vi "integral_ctrl_v7.vi"(4 "Lower limit":fxp<+/-,25,4>=-5.0, 5 "Upper limit":fxp<+/-,25,4>=5.0, 7 "Enable?":bool, 10 "Ki*Ts":fxp<+,16,0>, 11 "Input":fxp<+/-,25,4>) -> (3 "Output":fxp<+/-,25,4> format="%.23g")   [LabVIEW 2017, in "FPGA Controllers.lvlib"]
doc: "Integral controller implementation\nImplements: Ki/s in discrete time. (Ki*Ts) z / (z-1)\n\nAnti-windup limits can be specified as needed."
uses:
  FPGA Controllers.lvlib
  <vilib>/rvi/FXPMathLib/FxpMul/XNode/nifxpmath_Multiplier.xnode
  <vilib>/rvi/FXPMathLib/FxpAdd/XNode/nifxpmath_Add.xnode
  <vilib>/Platform/TimedLoop/XDataNode/XDataNode.xnode
  <vilib>/Platform/TimedLoop/XDataNode/nitl_modes.ctl
  <vilib>/Platform/TimedLoop/XDataNode/XDNodeRunTimeDep.lvlib
  <vilib>/Platform/TimedLoop/XDataNode/wakeup.ctl
  <vilib>/Platform/TimedLoop/XDataNode/timing_clust.ctl
  <vilib>/rvi/FXPMathLib/sim/FxpSim.dll
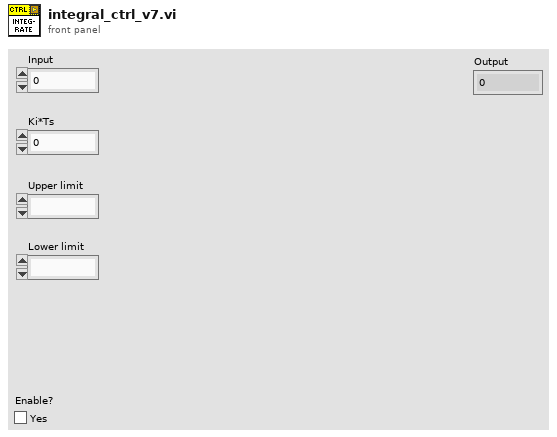
[diagram p1: front panel]
types:
  T1 = typedef "XDNodeRunTimeDep.lvlib/timing_clust.ctl" = cluster{"Expected End [f-1]":u64, "Actual End [f-1]":u64, "Finished Late? [f-1]":bool, "Expected End [i-1]":u64, "Actual End [i-1]":u64, "Finished Late? [i-1]":bool, "Expected Start [i]":u64, "Actual Start [i]":u64, "Expected Start [f]":u64, "Actual Start [f]":u64, "Source Name":string, "Structure Name":string, "Period":i64, "Deadline":i64, "Offset":i64, "Start":i64, "Priority":i32, "Timeout":i32, "Mode":T2, "Wakeup Reason":T3, "Error":errorcluster, "Source Type":string, "Secondary Source Type":string, "Global End Time":u64, "Global Start Time":u64, "Frame Duration":u64, "Iteration Duration":u64, "Assigned CPU":i32, "I/O Scan Engine Mode":u32}
  T2 = typedef "XDNodeRunTimeDep.lvlib/nitl_modes.ctl" = enum32{"No Change", "Process missed periods, maintain original phase", "Discard missed periods, maintain original phase", "Process missed periods, ignore original phase", "Discard missed periods, ignore original phase"}
  T3 = typedef "XDNodeRunTimeDep.lvlib/wakeup.ctl" = enum32{"Normal", "Aborted", "Asynchronous wakeup", "Timing source error", "Timed loop error", "Timeout"}
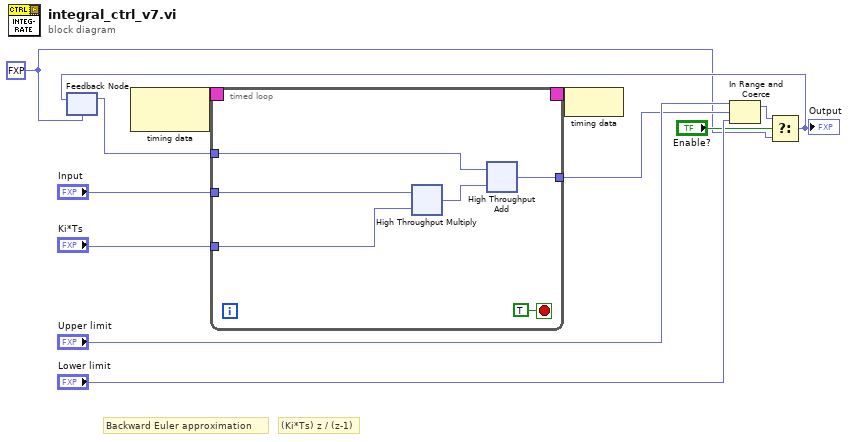
[diagram p0: block diagram]
diagram:
  w2 = fxp<+/-,25,4> 0.0 ("Input")
  # "(Ki*Ts) z / (z-1)"
  # "Backward Euler approximation"
  n1 = feedback #1(w2) -> (w4:fxp<+/-,25,4>)
  n2 = node-c288() -> (w6:T1)  [unwired: 1 in]
  n3 = timed-loop {
    timing: w6 -> [_]
    timing-out: [_] -> w5
    tunnel: "Ki*Ts" -> [w13]
    tunnel: w4 -> [w17]
    tunnel: "Input" -> [w18]
    tunnel: [w16] -> w7
    stop <- TRUE stop-if-true
    n4 = xnode ("High Throughput Multiply")("x"=w18, "y"=w13) -> ("x*y"=w15:fxp<+/-,25,4>)
    n5 = xnode ("High Throughput Add")("x"=w17, "y"=w15) -> ("x+y"=w16:fxp<+/-,25,4>)
  }
  n6 = node-c288(w5) -> ()
  n7 = In Range and Coerce(upper limit="Upper limit", x=w7, lower limit="Lower limit") -> (coerced(x)=w1:fxp<+/-,25,4>)  [unwired: 1 out]
  n8 = Select(t=w1, s="Enable?", f=w2) -> (s? t:f=w3:fxp<+/-,25,4>)
  "Output" <- w3
  n9 = feedback-in #1(w3) -> ()
